vi "Bytes at Port.vi"(0 "UART Driver in":refnum<class "UART Driver.lvclass">, 11 "error in":errorcluster) -> (4 "UART Driver out":refnum<class "UART Driver.lvclass">, 6 "Bytes at Input Buffer":u32, 15 "error out":errorcluster)   [LabVIEW 2012, in "UART_Host_Driver.lvlib" / "UART Driver.lvclass"]
uses:
  UART Driver.lvclass
  Typedefs/FPGA VI Reference.ctl
  UART Driver.lvclass/UART Driver.ctl
  <vilib>/Utility/error.llb/Error Cluster From Error Code.vi
  <vilib>/rvi/errors/niLvFpgaAdjustHostInterfaceError.vi
  <vilib>/rvi/interface/nirviMethod/nirviMethod.xnode
  UART_Host_Driver.lvlib
  <vilib>/FPGAPlugInAG/Dynamic/niLvFpga_ReadFifo_Dynamic.vi
  <vilib>/rvi/errors/niLvFpgaMergeErrorWithErrorCode.vi
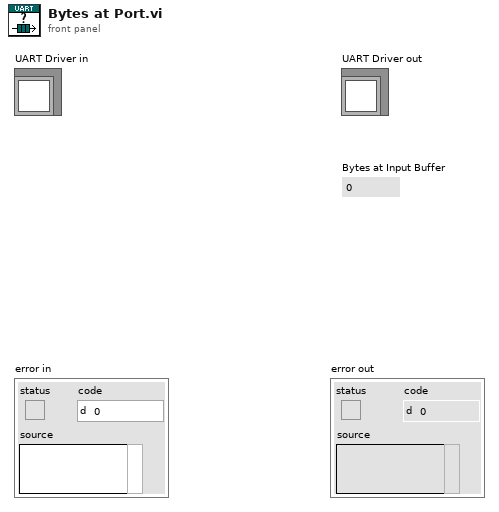
[diagram p1: front panel]
types:
  T1 = typedef "UART_Host_Driver.lvlib/FPGA VI Reference.ctl" = refnum<k20>
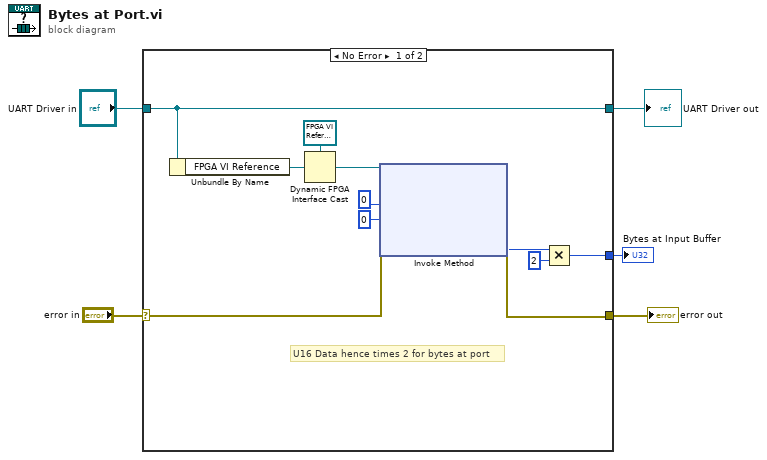
[diagram p0: block diagram]
diagram:
  n1 = case shown="No Error" "error in" {
    selector: "error in" -> [w12 w18]
    tunnel: [w11 w18] -> w4
    tunnel: [w16 w17] -> w2
    tunnel: "UART Driver in" -> [w16 w17]
    tunnel: [w9 _] -> w1
    frame No Error {
      # "U16 Data hence times 2 for bytes at port"
      n2 = Unbundle By Name(w16) -> ("FPGA VI Reference"=w15:refnum<k20>)
      n3 = Dynamic FPGA Interface Cast(Session In=T1 refnum ("FPGA VI Reference"), Type=w15) -> (Session Out=w13:T1)
      n4 = xnode "Invoke Method"("FPGA VI Reference In"=w13, "error in"=w12, "Number of Elements"=u32 0, "Timeout (ms)"=0) -> ("error out"=w11:errorcluster, "Elements Remaining"=w8:u32)  [unwired: 2 out]
      n5 = Multiply(x=w8, y=u32 2) -> (x*y=w9:u32)
    }
    frame Error {
    }
  }
  "error out" <- w4
  "UART Driver out" <- w2
  "Bytes at Input Buffer" <- w1
